vi "Write to File.vi"(8 "error in (no error)":errorcluster, 11 "Report.lvclass":refnum<class "Wind Report.lvclass">) -> (0 "error out":errorcluster, 3 "Report out":refnum<class "Wind Report.lvclass">)   [LabVIEW 2009, in "Wind Report.lvclass"]
doc: "This dynamic dispatch VI is overriden by the child classes.\n\nAAL 9/09"
uses:
  Wind Report.lvclass
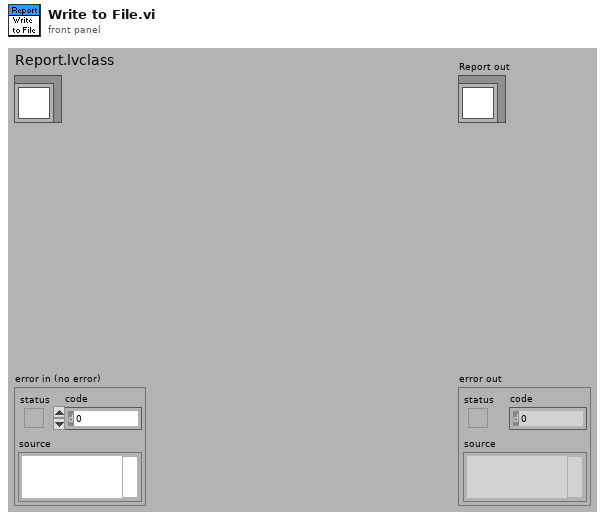
[diagram p1: front panel]
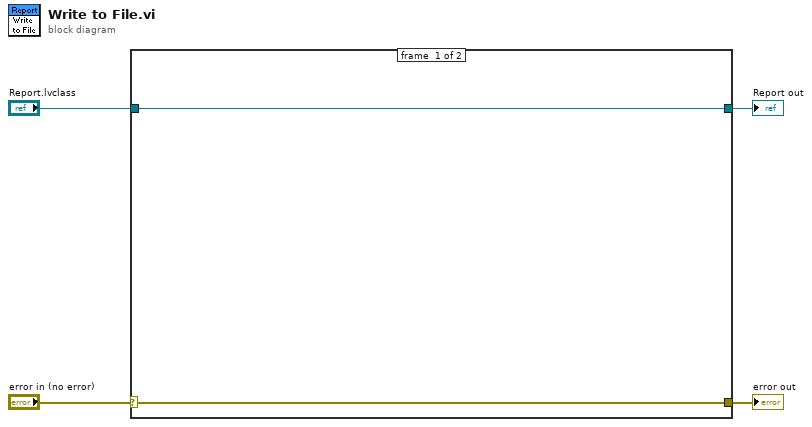
[diagram p0: block diagram]
diagram:
  n1 = case shown="No Error" "error in (no error)" {
    selector: "error in (no error)" -> [w5 w8]
    tunnel: [w5 w8] -> w3
    tunnel: [w6 w7] -> w2
    tunnel: "Report.lvclass" -> [w6 w7]
    frame #0 {
    }
    frame #1 {
    }
  }
  "error out" <- w3
  "Report out" <- w2
